vi "电源管理UI.vi"() -> ()   [LabVIEW 2016, in "PLC.lvlib"]
uses:
  PLC.lvlib
  <vilib>/Utility/miscctls.llb/LVPointTypeDef.ctl
panel:
  in  "看门狗启用":bool
  out "R123":i16 caption="看门狗设置"
  out "R56":i16 caption="看门狗计时器"
  in  "自动运行启动参数":T1
  # "看门狗设置"
  # "说明：\n系统模式处于维护模式时，仪器电源自动打开；\n系统模式处于常规模式/质控模式/应急模式下，周期启动时，仪器电源自动打开；"
  # "S"
  # "S"
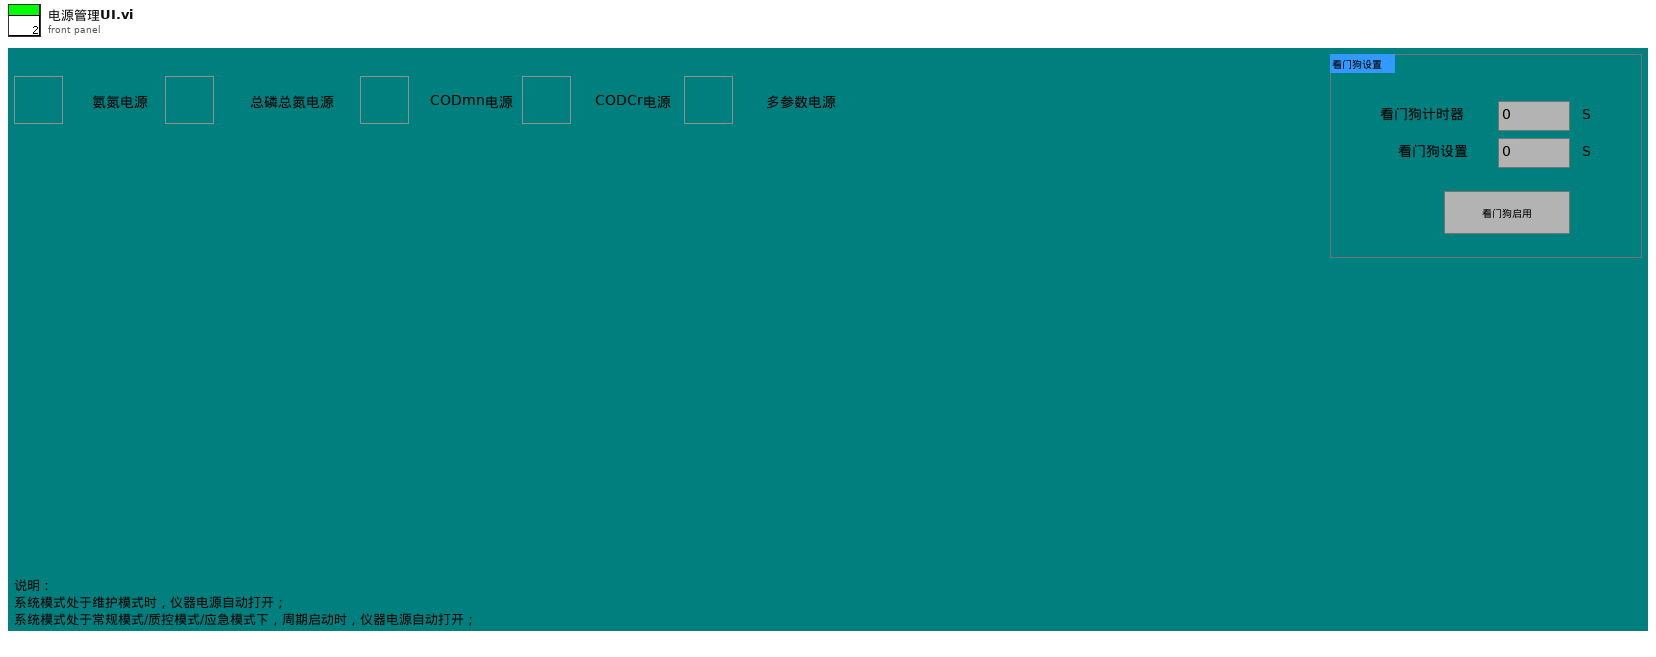
[diagram p1: front panel]
types:
  T1 = cluster{"氨氮":bool, "总磷总氮":bool, "CODmn":bool, "CODCr":bool, "多参数":bool}
  T2 = typedef "LVPointTypeDef.ctl" = cluster{"Horizontal":i16, "Vertical":i16}
  T3 = cluster{"R100":i16, "R101":i16, "R102":i16, "R103":i16, "R104":i16, "R105":i16, "R106":i16, "R107":i16, "R108":i16, "R109":i16, "R110":i16, "R111":i16, "R112":i16, "R113":i16, "R114":i16, "R115":i16, "R116":i16, "R117":i16, "R118":i16, "R119":i16, "R120":i16, "R121":i16, "R122":i16, "R123":i16, "R124":i16}
  T4 = cluster{"R0":i16, "R1":i16, "R2":i16, "R3":i16, "R4":i16, "R5":i16, "R6":i16, "R7":i16, "R8":i16, "R9":i16, "R10":i16, "R11":i16, "R12":i16, "R13":i16, "R14":i16, "R15":i16, "R16":i16, "R17":i16, "R18":i16, "R19":i16, "R20":i16, "R21":i16, "R22":i16, "R23":i16, "R24":i16, "R25":i16, "R26":i16, "R27":i16, "R28":i16, "R29":i16, "R30":i16, "R31":i16, "R32":i16, "R33":i16, "R34":i16, "R35":i16, "R36":i16, "R37":i16, "R38":i16, "R39":i16, "R40":i16, "R41":i16, "R42":i16, "R43":i16, "R44":i16, "R45":i16, "R46":i16, "R47":i16, "R48":i16, "R49":i16, "R50":i16, "R51":i16, "R52":i16, "R53":i16, "R54":i16, "R55":i16, "R56":i16}
  T5 = cluster{"命令":string, "数据":cluster{"starting address":u16, "holding register values":u16[]}}
  T6 = cluster{"命令":string, "data":cluster{"starting address":u16, "coil values":bool[]}}
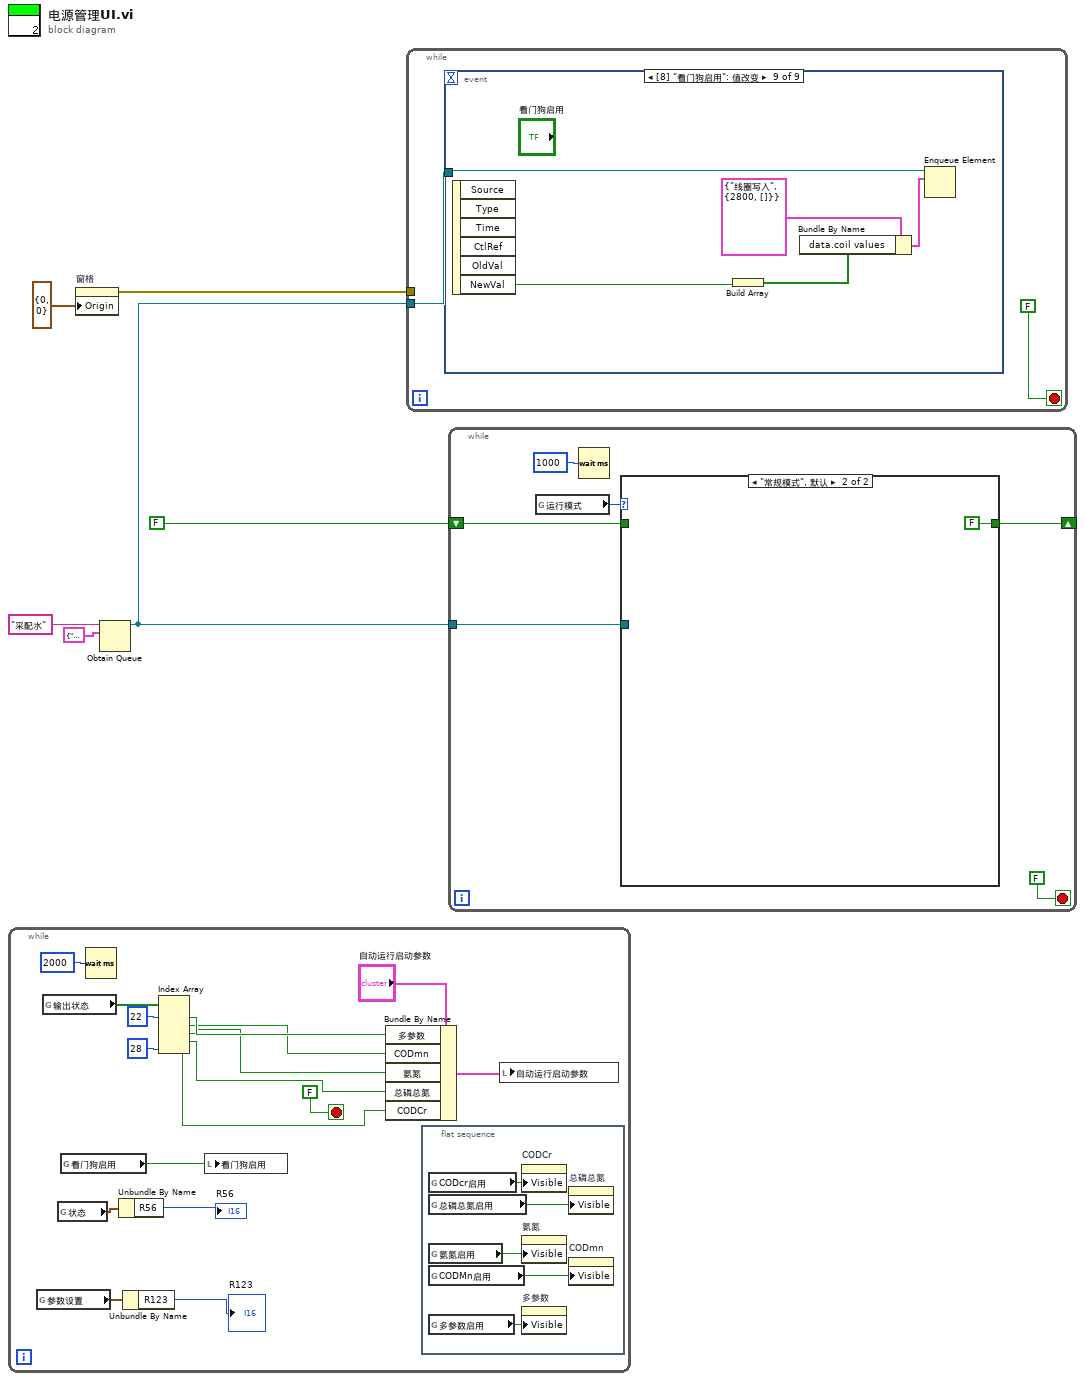
[diagram p0: block diagram]
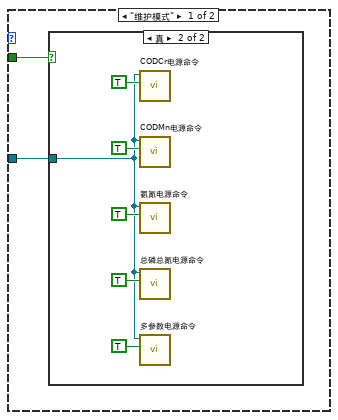
[diagram p2: hidden frame]
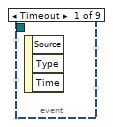
[diagram p4: hidden frame]
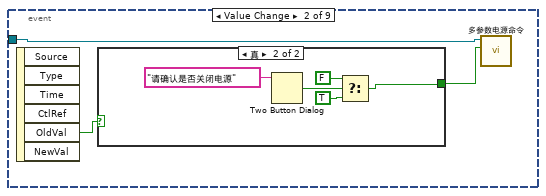
[diagram p5: hidden frame]
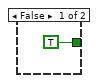
[diagram p6: hidden frame]
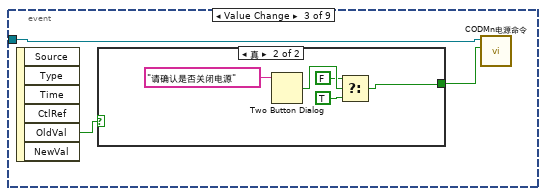
[diagram p7: hidden frame]
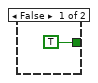
[diagram p8: hidden frame]
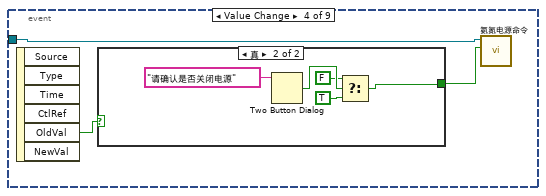
[diagram p9: hidden frame]
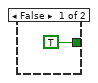
[diagram p10: hidden frame]
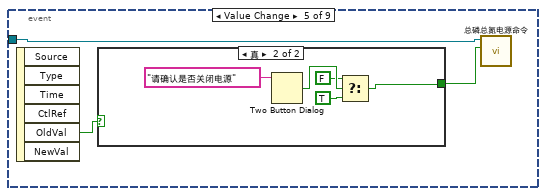
[diagram p11: hidden frame]
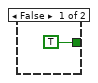
[diagram p12: hidden frame]
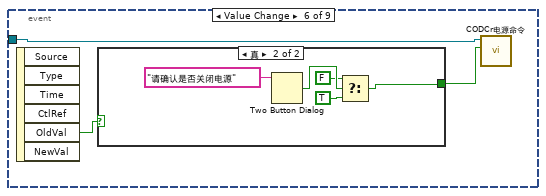
[diagram p13: hidden frame]
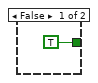
[diagram p14: hidden frame]
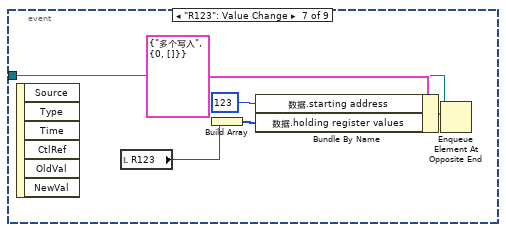
[diagram p15: hidden frame]
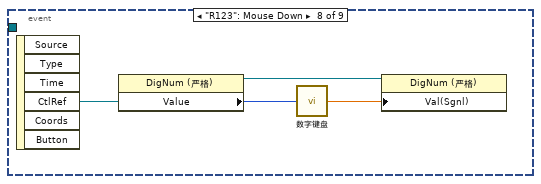
[diagram p16: hidden frame]
diagram:
  n1 = while {
    stop <- FALSE stop-if-true
    n2 = global read "采配水全局变量.vi" "参数设置"() -> (w9:T3)
    n3 = global read "采配水全局变量.vi" "输出状态"() -> (w21:bool[])
    n4 = global read "采配水全局变量.vi" "状态"() -> (w11:T4)
    n5 = global read "采配水全局变量.vi" "看门狗启用"() -> (w7:bool)
    n6 = Wait (ms)(milliseconds to wait=u32 2000 ("等待时间（毫秒）")) -> ()  [unwired: 1 out]
    n7 = Unbundle By Name(w11) -> ("R56"=→"R56":i16)
    n8 = Unbundle By Name(w9) -> ("R123"=→"R123":i16)
    n9 = Index Array(array=w21, index #1=22 ("索引"), index #5=28 ("索引")) -> (element #1=w17:bool, element #2=w16:bool, element #3=w15:bool, element #4=w14:bool, element #5=w13:bool)  [unwired: 3 in]
    n10 = local write "看门狗启用"(w7) -> ()
    n11 = Bundle By Name(cluster="自动运行启动参数", "多参数"=w17, "CODmn"=w16, "氨氮"=w15, "总磷总氮"=w14, "CODCr"=w13) -> (w12:T1)
    n12 = flat-sequence {
      frame #0 {
        n13 = global read "系统设置全局变量.vi" "CODcr启用"() -> (w28:bool)
        n14 = global read "系统设置全局变量.vi" "总磷总氮启用"() -> (w24:bool)
        n15 = global read "系统设置全局变量.vi" "氨氮启用"() -> (w26:bool)
        n16 = global read "系统设置全局变量.vi" "CODMn启用"() -> (w27:bool)
        n17 = global read "系统设置全局变量.vi" "多参数启用"() -> (w25:bool)
        n18 = property on="CODCr" class="Bool (严格)"("Visible"=w28) -> ()  [unwired: 2 in, 2 out]
        n19 = property on="氨氮" class="Bool (严格)"("Visible"=w26) -> ()  [unwired: 2 in, 2 out]
        n20 = property on="多参数" class="Bool (严格)"("Visible"=w25) -> ()  [unwired: 2 in, 2 out]
        n21 = property on="总磷总氮" class="Bool (严格)"("Visible"=w24) -> ()  [unwired: 2 in, 2 out]
        n22 = property on="CODmn" class="Bool (严格)"("Visible"=w27) -> ()  [unwired: 2 in, 2 out]
      }
    }
    n23 = local write "自动运行启动参数"(w12) -> ()
  }
  n24 = property on="窗格" class="Pane"("Origin"=T2 {"Horizontal"=0, "Vertical"=0} ("原点")) -> (error out=w3:errorcluster)  [unwired: 2 in, 1 out]
  n25 = Obtain Queue(name (unnamed)="采配水" ("名称（未命名）"), element data type=cluster{"命令":string, "数据":variant} {"命令"="", "数据"=variant}) -> (queue out=w2:refnum<queue>)  [unwired: 3 in, 2 out]
  n26 = while {
    tunnel: w2 -> [w29]
    tunnel: w3 -> [_]
    stop <- FALSE stop-if-true
    n27 = event shown="[8] \"看门狗启用\": 值改变" {
      selector: _ -> [_ _ _ _ _ _ _ _ _]
      dyn-events: _ -> [_ _ _ _ _ _ _ _ _]
      timeout: _ -> [_ _ _ _ _ _ _ _ _]
      tunnel: w29 -> [_ w33 w42 w51 w60 w69 w77 _ w86]
      event Timeout {
        n28 = event-data() -> ()  [unwired: 1 in, 3 out]
      }
      event "自动运行启动参数.多参数": Value Change {
        n29 = event-data() -> ("OldVal"=w32:bool)  [unwired: 1 in, 5 out]
        n30 = case shown="真" w32 {
          tunnel: [TRUE ("T button?") w35] -> w31
          frame False {
          }
          frame True {
            n31 = Two Button Dialog(message="请确认是否关闭电源" ("消息")) -> (T button?=w38:bool)  [unwired: 2 in]
            n32 = Select(t=FALSE, s=w38, f=TRUE ("T button?")) -> (s? t:f=w35:bool)
          }
        }
        n33 = call "多参数电源命令.vi"("通电/断电"=w31, "队列"=w33) -> ()  [unwired: 9 in, 1 out]
      }
      event "自动运行启动参数.CODmn": Value Change {
        n34 = event-data() -> ("OldVal"=w41:bool)  [unwired: 1 in, 5 out]
        n35 = case shown="真" w41 {
          tunnel: [TRUE ("T button?") w44] -> w40
          frame False {
          }
          frame True {
            n36 = Two Button Dialog(message="请确认是否关闭电源" ("消息")) -> (T button?=w47:bool)  [unwired: 2 in]
            n37 = Select(t=FALSE, s=w47, f=TRUE ("T button?")) -> (s? t:f=w44:bool)
          }
        }
        n38 = call "CODMn电源命令.vi"("通电/断电"=w40, "队列"=w42) -> ()  [unwired: 9 in, 1 out]
      }
      event "自动运行启动参数.氨氮": Value Change {
        n39 = event-data() -> ("OldVal"=w50:bool)  [unwired: 1 in, 5 out]
        n40 = case shown="真" w50 {
          tunnel: [TRUE ("T button?") w53] -> w49
          frame False {
          }
          frame True {
            n41 = Two Button Dialog(message="请确认是否关闭电源" ("消息")) -> (T button?=w56:bool)  [unwired: 2 in]
            n42 = Select(t=FALSE, s=w56, f=TRUE ("T button?")) -> (s? t:f=w53:bool)
          }
        }
        n43 = call "氨氮电源命令.vi"("通电/断电"=w49, "队列"=w51) -> ()  [unwired: 9 in, 1 out]
      }
      event "自动运行启动参数.总磷总氮": Value Change {
        n44 = event-data() -> ("OldVal"=w59:bool)  [unwired: 1 in, 5 out]
        n45 = case shown="真" w59 {
          tunnel: [TRUE ("T button?") w62] -> w58
          frame False {
          }
          frame True {
            n46 = Two Button Dialog(message="请确认是否关闭电源" ("消息")) -> (T button?=w65:bool)  [unwired: 2 in]
            n47 = Select(t=FALSE, s=w65, f=TRUE ("T button?")) -> (s? t:f=w62:bool)
          }
        }
        n48 = call "总磷总氮电源命令.vi"("通电/断电"=w58, "队列"=w60) -> ()  [unwired: 9 in, 1 out]
      }
      event "自动运行启动参数.CODCr": Value Change {
        n49 = event-data() -> ("OldVal"=w68:bool)  [unwired: 1 in, 5 out]
        n50 = case shown="真" w68 {
          tunnel: [TRUE ("T button?") w71] -> w67
          frame False {
          }
          frame True {
            n51 = Two Button Dialog(message="请确认是否关闭电源" ("消息")) -> (T button?=w74:bool)  [unwired: 2 in]
            n52 = Select(t=FALSE, s=w74, f=TRUE ("T button?")) -> (s? t:f=w71:bool)
          }
        }
        n53 = call "CODCr电源命令.vi"("通电/断电"=w67, "队列"=w69) -> ()  [unwired: 9 in, 1 out]
      }
      event "R123": Value Change {
        n54 = event-data() -> ()  [unwired: 1 in, 6 out]
        n55 = local read "R123"() -> (w76:i16)
        n56 = Build Array(w76) -> (w81:i16[])
        n57 = Bundle By Name(cluster=T5 {"命令"="多个写入", "数据"={"starting address"=0, "holding register values"=[]}} ("元素"), "数据.starting address"=u16 123, "数据.holding register values"=w81) -> (w80:T5)
        n58 = Enqueue Element At Opposite End(queue=w77, element=w80) -> ()  [unwired: 2 in, 3 out]
      }
      event "R123": Mouse Down {
        n59 = event-data() -> ("CtlRef"=w82:refnum<vi>)  [unwired: 1 in, 5 out]
        n60 = property class="DigNum (严格)"(reference=w82) -> (reference out=w84:refnum<vi>, "Value"=w85:i16)  [unwired: 1 in, 1 out]
        n61 = call "数字键盘.vi"("OldNumber"=w85) -> ("NewNumber"=w83:sgl)
        n62 = property class="DigNum (严格)"(reference=w84, "Val(Sgnl)"=w83) -> ()  [unwired: 1 in, 2 out]
      }
      event "看门狗启用": Value Change {
        n63 = event-data() -> ("NewVal"=w88:bool)  [unwired: 1 in, 5 out]
        n64 = Build Array(w88) -> (w87:bool[])
        n65 = Bundle By Name(cluster=T6 {"命令"="线圈写入", "data"={"starting address"=2800, "coil values"=[]}} ("元素"), "data.coil values"=w87) -> (w89:T6)
        n66 = Enqueue Element(queue=w86, element=w89) -> ()  [unwired: 2 in, 3 out]
      }
    }
  }
  n67 = while {
    tunnel: w2 -> [w94]
    shift-right: [w91] -> _
    shift-left: FALSE -> [w92]
    stop <- FALSE stop-if-true
    n68 = global read "系统设置全局变量.vi" "运行模式"() -> (w93:enum16{"维护模式", "常规模式", "应急模式", "质控模式"})
    n69 = Wait (ms)(milliseconds to wait=u32 1000 ("等待时间（毫秒）")) -> ()  [unwired: 1 out]
    n70 = case shown="\"常规模式\", 默认" w93 {
      tunnel: w94 -> [w98 _]
      tunnel: w92 -> [w97 _]
      tunnel: [_ FALSE] -> w91
      frame "维护模式" {
        n71 = case shown="真" w97 {
          tunnel: w98 -> [_ w99]
          frame False {
          }
          frame True {
            n72 = call "CODCr电源命令.vi"("通电/断电"=TRUE, "队列"=w99) -> ()  [unwired: 9 in, 1 out]
            n73 = call "CODMn电源命令.vi"("通电/断电"=TRUE, "队列"=w99) -> ()  [unwired: 9 in, 1 out]
            n74 = call "氨氮电源命令.vi"("通电/断电"=TRUE, "队列"=w99) -> ()  [unwired: 9 in, 1 out]
            n75 = call "总磷总氮电源命令.vi"("通电/断电"=TRUE, "队列"=w99) -> ()  [unwired: 9 in, 1 out]
            n76 = call "多参数电源命令.vi"("通电/断电"=TRUE, "队列"=w99) -> ()  [unwired: 9 in, 1 out]
          }
        }
      }
      frame "常规模式", Default {
      }
    }
  }
